vi "X Y to galvo signal.vi"(10 "initial y":u16=32768, 11 "initial x":u16=32768) -> (3 "array":u32[](array[numeric]))   [LabVIEW 2015]
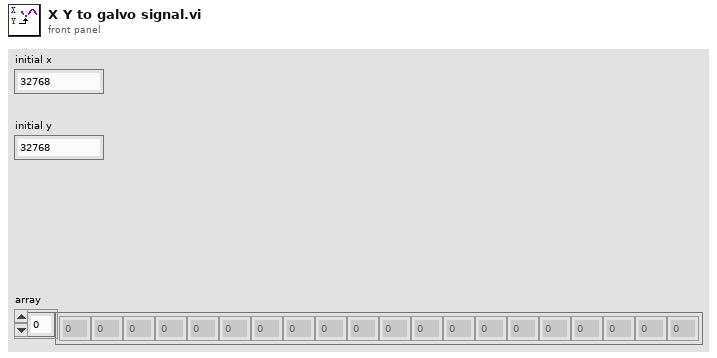
[diagram p1: front panel]
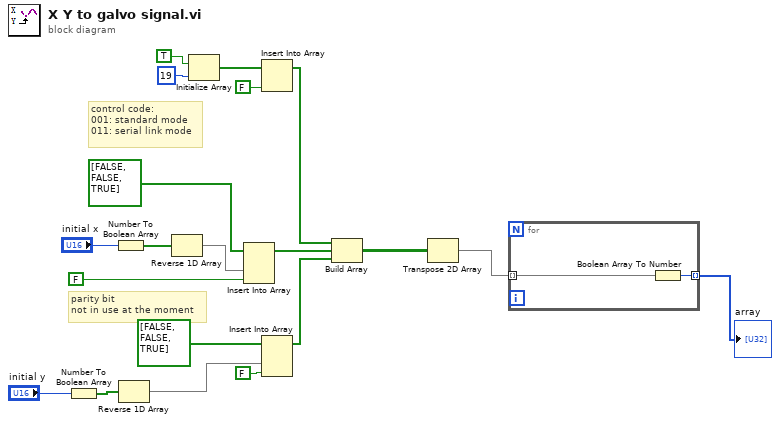
[diagram p0: block diagram]
diagram:
  # "parity bit\nnot in use at the moment"
  # "control code:\n001: standard mode\n011: serial link mode"
  n1 = Number To Boolean Array(number="initial y") -> (Boolean array=w19:bool[])
  n2 = Number To Boolean Array(number="initial x") -> (Boolean array=w10:bool[])
  n3 = Reverse 1D Array(array=w19) -> (reversed array=w17:bool[])
  n4 = Reverse 1D Array(array=w10) -> (reversed array=w8:bool[])
  n5 = Initialize Array(TRUE ("element"), 19 ("dimension size")) -> (w13:bool[])
  n6 = Insert Into Array(array=bool[] [FALSE, FALSE, TRUE] ("Array"), new element #1=w8, new element #2=FALSE) -> (w6:bool[])  [unwired: 1 in]
  n7 = Insert Into Array(array=w13, new element=FALSE ("element")) -> (w12:bool[])  [unwired: 1 in]
  n8 = Insert Into Array(array=bool[] [FALSE, FALSE, TRUE] ("Array"), new element #1=w17, new element #2=FALSE) -> (w5:bool[])  [unwired: 1 in]
  n9 = Build Array(w12, w6, w5) -> (w4:bool[][])
  n10 = Transpose 2D Array(2D array=w4) -> (transposed array=w3:bool[][])
  n11 = for {
    tunnel: w3 -> [w22] mode=indexing
    tunnel: [w21] -> w2 mode=indexing
    n12 = Boolean Array To Number(Boolean array=w22) -> (number=w21:u32)
  }
  "array" <- w2
